vi "Csatornák létrehozása 6.0.vi"(8 "error in":errorcluster, 11 "Analog data in":T3) -> (0 "error out":errorcluster, 3 "Analog data out":T3)   [LabVIEW 2014]
uses:
  Analog data.ctl
  Analog Input Cluster.ctl
  Analog Result Cluster.ctl
panel:
  in  "NI Analog Input":T1 {"Analog Result"."Számolt NTC hõmérséklet" format="%.3g"; "Analog Result"."15V" format="%.3g"; "Analog Result"."Elvárt NTC ellenállás" format="%.3g"; "Analog Result"."48V" format="%.3g"; "Analog Result"."Hõmérséklet" format="%.3g"; "Analog Result"."Szigetelési ellenállás" format="%.3g"; "Analog Result"."NTC ellenállás" format="%.3g"; "Analog Result"."Szenzor ellenállás" format="%.3g"}
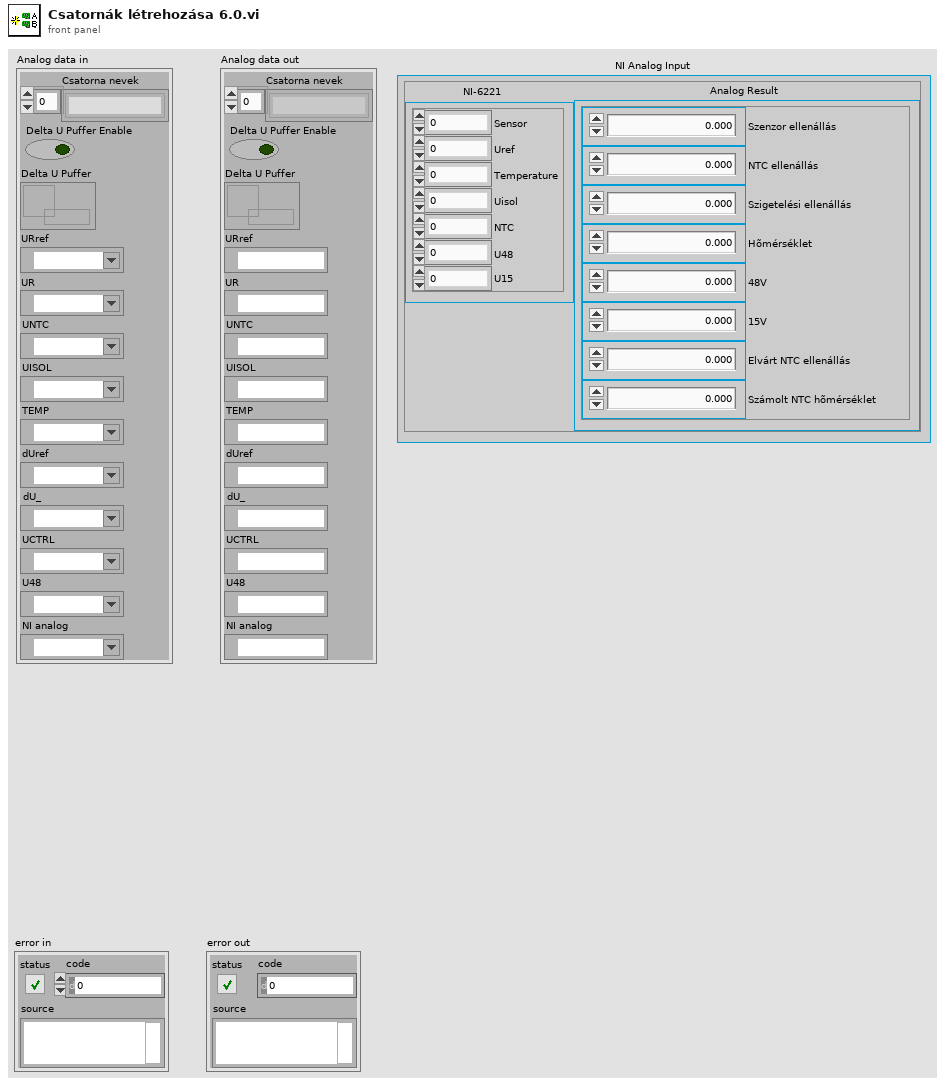
[diagram p1: front panel]
types:
  T1 = typedef "Analog Input Cluster.ctl" = cluster{"NI-6221":cluster{"Sensor":dbl, "Uref":dbl, "Temperature":dbl, "Uisol":dbl, "NTC":dbl, "U48":dbl, "U15":dbl}, "Analog Result":T2}
  T2 = typedef "Analog Result Cluster.ctl" = cluster{"Szenzor ellenállás":dbl, "NTC ellenállás":dbl, "Szigetelési ellenállás":dbl, "Hõmérséklet":dbl, "48V":dbl, "15V":dbl, "Elvárt NTC ellenállás":dbl, "Számolt NTC hõmérséklet":dbl}
  T3 = typedef "Analog data.ctl" = cluster{"Csatorna nevek":string[], "Delta U Puffer Enable":bool, "Delta U Puffer":refnum<queue>, "URref":refnum<k21>, "UR":refnum<k21>, "UNTC":refnum<k21>, "UISOL":refnum<k21>, "TEMP":refnum<k21>, "dUref":refnum<k21>, "dU_":refnum<k21>, "UCTRL":refnum<k21>, "U48":refnum<k21>, "NI analog":refnum<k21>}
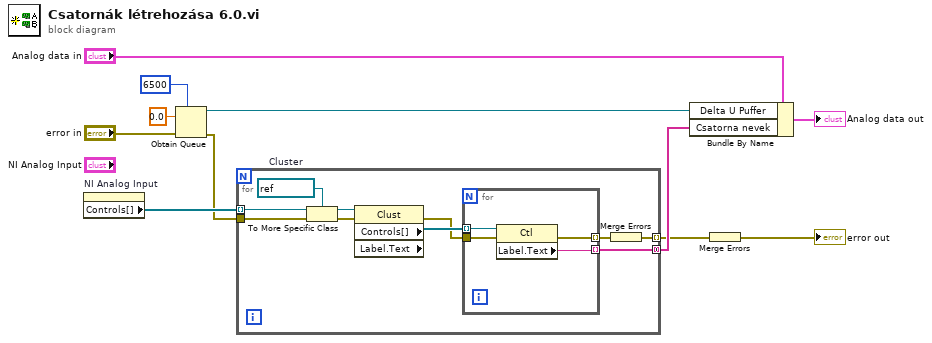
[diagram p0: block diagram]
diagram:
  n1 = property on="NI Analog Input" class="Clust (strict)"() -> ("Controls[]"=w5:refnum<vi>[])  [unwired: 2 in, 2 out]
  n2 = Obtain Queue(max queue size (-1, unlimited)=6500, element data type=0.0, error in (no error)="error in") -> (queue out=w6:refnum<queue>, error out=w3:errorcluster)  [unwired: 2 in, 1 out]
  n3 = for {
    tunnel: w5 -> [w18] mode=indexing
    tunnel: [w17] -> w4 mode=concatenating
    tunnel: w3 -> [w16]
    tunnel: [w13] -> w2 mode=indexing
    w21 = refnum<vi> refnum  # Cluster
    n4 = To More Specific Class(target class=w21, reference=w18, error in=w16) -> (specific class reference=w20:refnum<vi>, error out=w15:errorcluster)
    n5 = property class="Clust" props=["Controls[]", "Label", "Text"](reference=w20, error in=w15) -> (error out=w14:errorcluster, "Controls[]"=w19:refnum<vi>[])  [unwired: 2 out]
    n6 = for {
      tunnel: w19 -> [w25] mode=indexing
      tunnel: [w24] -> w17 mode=indexing
      tunnel: w14 -> [w23]
      tunnel: [w22] -> w12 mode=indexing
      n7 = property class="Ctl"(reference=w25, error in=w23) -> (error out=w22:errorcluster, "Label.Text"=w24:string)  [unwired: 1 out]
    }
    n8 = Merge Errors(w12) -> (w13:errorcluster)
  }
  n9 = Bundle By Name(cluster="Analog data in", "Delta U Puffer"=w6, "Csatorna nevek"=w4) -> (→"Analog data out":T3)
  n10 = Merge Errors(w2) -> (→"error out":errorcluster)
